vi "Speak.vi"(0 "voice":i32, 1 "GetVoices":refnum<k7>, 2 "GetAudioOutputs":refnum<k7>, 3 "SpeechLib.ISpeechVoice (In)":refnum<k7>, 5 "audio device":i32, 7 "Speech Rate":i32, 9 "Volume Control":i32, 11 "error in":errorcluster, 12 "Flags":i32, 13 "String":string) -> (4 "SpeechLib.ISpeechVoice (Out)":refnum<k7>, 6 "GetAudioOutputs (out)":refnum<k7>, 8 "GetVoices (out)":refnum<k7>, 15 "error out (no error)":errorcluster)   [LabVIEW 2018]
doc: "This SubVI calls the speak command from the Microsoft Speech SDK 5.1 software."
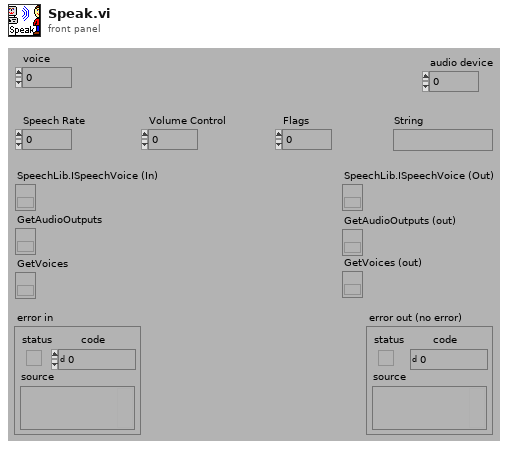
[diagram p1: front panel]
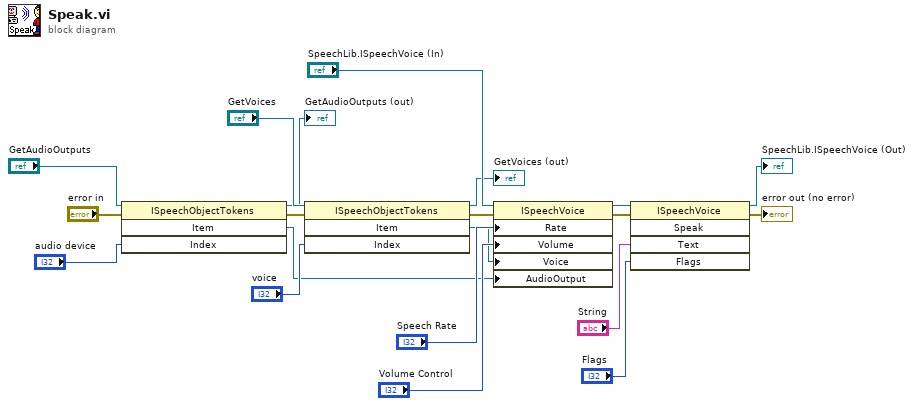
[diagram p0: block diagram]
diagram:
  n1 = invoke class="ISpeechObjectTokens" method="Item"(reference="GetAudioOutputs", error in="error in", "Index"="audio device") -> (reference out=→"GetAudioOutputs (out)":refnum<k7>, error out=w2:errorcluster, "Item"=w5:refnum<k7>)  [unwired: 1 in, 1 out]
  n2 = invoke class="ISpeechObjectTokens" method="Item"(reference="GetVoices", error in=w2, "Index"="voice") -> (reference out=→"GetVoices (out)":refnum<k7>, error out=w1:errorcluster, "Item"=w6:refnum<k7>)  [unwired: 1 in, 1 out]
  n3 = property class="ISpeechVoice"(reference="SpeechLib.ISpeechVoice (In)", error in=w1, "Rate"="Speech Rate", "Volume"="Volume Control", "Voice"=w6, "AudioOutput"=w5) -> (reference out=w4:refnum<k7>, error out=w3:errorcluster)
  n4 = invoke class="ISpeechVoice" method="Speak"(reference=w4, error in=w3, "Text"="String", "Flags"="Flags") -> (reference out=→"SpeechLib.ISpeechVoice (Out)":refnum<k7>, error out=→"error out (no error)":errorcluster)  [unwired: 1 in, 3 out]
